vi "Thermistor 4Wire Get Low Power.vi"(8 "error in (no error)":errorcluster {"code" format="%.0x"}, 9 "ValBufferSize":i32=2048, 10 "ChannelList":string, 11 "instrument handle":refnum<k15>) -> (0 "error out":errorcluster {"code" format="%.0x"}, 1 "ValActualSize":i32, 2 "Val":u16[](array[numeric]), 3 "instrument handle out":refnum<k15>)   [LabVIEW 2020, in "Keysight DAQ970.lvlib"]
doc: "Gets the low power enabled state of the specified channelList or current scan list if parameter is empty."
uses:
  Keysight DAQ970.lvlib
  KtDAQ970.dll
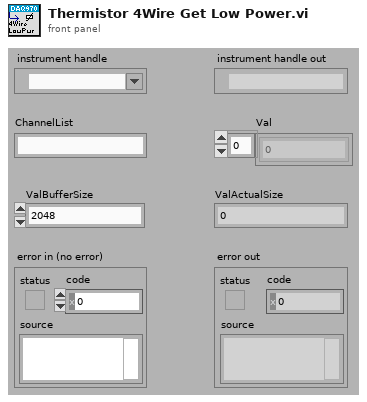
[diagram p1: front panel]
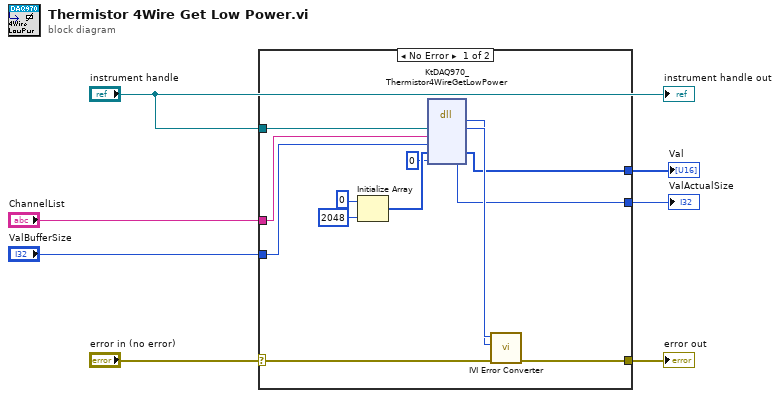
[diagram p0: block diagram]
diagram:
  n1 = case shown="No Error" "error in (no error)" {
    selector: "error in (no error)" -> [w17 w21]
    tunnel: [w16 w21] -> w7
    tunnel: "instrument handle" -> [w20 _]
    tunnel: "ChannelList" -> [w15 _]
    tunnel: "ValBufferSize" -> [w14 _]
    tunnel: [w10 _] -> w2
    tunnel: [w8 _] -> w1
    frame No Error {
      n2 = Initialize Array(u16 0 ("element"), 2048 ("dimension size")) -> (w13:u16[])
      n3 = dll-call lib="KtDAQ970**.dll" fn="KtDAQ970_Thermistor4WireGetLowPower"("Vi"=w20, "ChannelList"=w15, "ValBufferSize"=w14, "Val"=w13, "ValActualSize"=0) -> (w18:i32, "Vi"=w19:u32, "Val"=w10:u16[], "ValActualSize"=w8:i32)  [unwired: 5 in, 2 out]
      n4 = call "IVI Error Converter.vi"("error in (no error)"=w17, "IVI error code (0)"=w18, "instrument handle"=w19) -> ("error out"=w16:errorcluster)  [unwired: 7 in, 1 out]
    }
    frame Error {
    }
  }
  "error out" <- w7
  "Val" <- w2
  "ValActualSize" <- w1
  "instrument handle out" <- "instrument handle"
